vi "Load Configuration.vi"(8 "error in":errorcluster) -> (0 "error out":errorcluster, 3 "Theme Config out":refnum<class "Theme Config.lvclass">)   [LabVIEW 2021, in "Theme Config.lvclass"]
doc: "Load the configuration from file; if it doesn't exist, go ahead and create it so it can be referenced in the future.\n\nThis will allow persistence of the Material File in the editor and the Last Theme Mod implemented.\n\n<b>Code Developed By:</b>\nDaniel Coons\nTechnology Service Corporation\nwww.tsc.com/atcs"
uses:
  Theme Config.lvclass
  C:/Program Files/National Instruments/LabVIEW 2026/vi.lib/JDP Science/JSONtext/Config Files/Config File.lvclass
  Theme Serializer/Theme Serializer.lvclass
  C:/Program Files/National Instruments/LabVIEW 2026/vi.lib/JDP Science/JSONtext/LVClass Serializer/JSONtext LVClass Serializer.lvclass
  Theme Config.lvclass/Theme Config.ctl
  <vilib>/JDP Science/JSONtext/Config Files/Config File.lvclass/Config File.ctl
  3b317bd2-2840-4331-bfb7-99d377f3c52f.vi
  <vilib>/JDP Science/JSONtext/JSON text to Variant.vi
  <vilib>/JDP Science/JSONtext/Config Files/Config File.lvclass
  <vilib>/JDP Science/JSONtext/JSONtext.lvlib
  Material SubVIs/Material SubVIs.lvlib
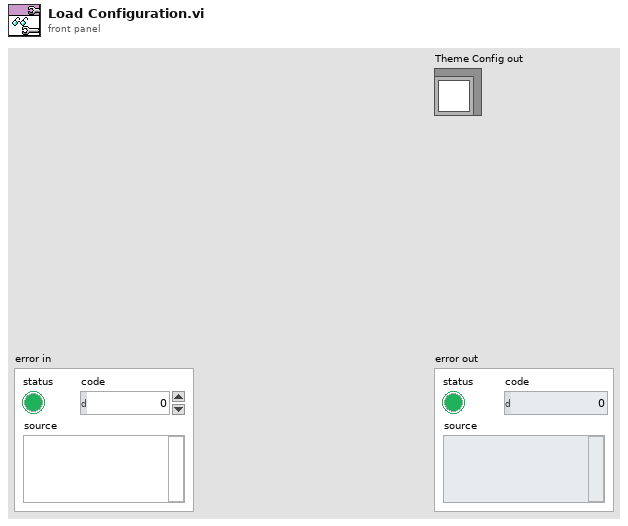
[diagram p1: front panel]
types:
  T1 = enum16{"open", "replace", "create", "open or create", "replace or create", "replace or create with confirmation"}
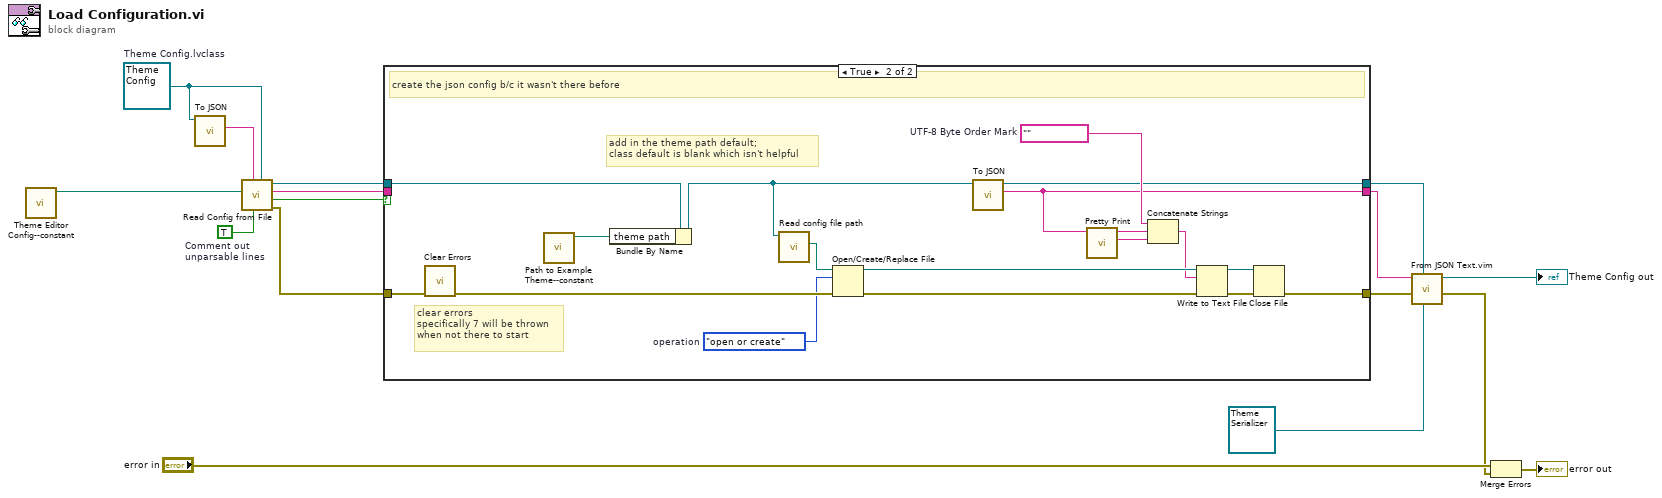
[diagram p0: block diagram]
diagram:
  w11 = TRUE  # Comment out unparsable lines
  w14 = refnum<class "Theme Config.lvclass"> refnum  # Theme Config.lvclass
  n1 = call "Theme Editor Config--constant.vi"() -> ("Button Editor Config"=w12:path)  [unwired: 11 in]
  n2 = call "To JSON.vi"("Theme Config in"=w14) -> ("JSON"=w13:string)  [unwired: 8 in, 2 out]
  n3 = call <vilib>:"Read Config from File.vi"("Config File (type)"=w14, "Comment out unparsable lines"=w11, "Template (JSON Object)"=w13, "config file path"=w12) -> ("error out"=w9:errorcluster, "Template Used (file missing or corrupted)"=w10:bool, "<JSON>Config"=w8:string, "Config File"=w7:refnum<class "Theme Config.lvclass">)  [unwired: 4 in]
  n4 = case shown="True" w10 {
    tunnel: w9 -> [w19 w37]
    tunnel: w8 -> [w18 _]
    tunnel: w7 -> [w17 w36]
    tunnel: [w17 w21] -> w4
    tunnel: [w18 w20] -> w5
    tunnel: [w19 w26] -> w6
    frame False {
    }
    frame True {
      w23 = T1."open or create"  # operation
      w30 = "﻿"  # UTF-8 Byte Order Mark
      # "add in the theme path default;\nclass default is blank which isn't helpful"
      # "clear errors\nspecifically 7 will be thrown\nwhen not there to start"
      # "create the json config b/c it wasn't there before"
      n5 = call <vilib>:"Clear Errors.vi"("error in (no error)"=w37) -> ("error out"=w24:errorcluster)  [unwired: 5 in, 1 out]
      n6 = call "Path to Example Theme--constant.vi"() -> ("Path to Example Theme"=w25:path)  [unwired: 11 in]
      n7 = Bundle By Name(cluster=w36, "theme path"=w25) -> (w22:refnum<class "Theme Config.lvclass">)
      n8 = call <vilib>:"Read config file path.vi"("Config File in"=w22) -> ("config file path"=w35:path)  [unwired: 10 in]
      n9 = Open/Create/Replace File(file path (use dialog)=w35, error in=w24, operation (0:open)=w23) -> (refnum out=w33:refnum<file>, error out=w34:errorcluster)  [unwired: 3 in, 1 out]
      n10 = call "To JSON.vi"("Theme Config in"=w22) -> ("JSON"=w20:string, "Theme Config out"=w21:refnum<class "Theme Config.lvclass">)  [unwired: 8 in, 1 out]
      n11 = call <vilib>:"Pretty Print.vi"("JSON"=w20) -> ("Rest of Input String"=w32:string, "<JSON>"=w31:string)  [unwired: 8 in, 1 out]
      n12 = Concatenate Strings(w30, w31, w32) -> (w29:string)
      n13 = Write to Text File(file (use dialog)=w33, text=w29, error in=w34) -> (refnum out=w27:refnum<file>, error out=w28:errorcluster)  [unwired: 1 in, 1 out]
      n14 = Close File(refnum=w27, error in=w28) -> (error out=w26:errorcluster)  [unwired: 1 out]
    }
  }
  n15 = call "From JSON Text.vim"("LVClass Serializer"=refnum<class "Theme Serializer.lvclass"> refnum ("Theme Serializer.lvclass"), "Data Type and Default Value"=w4, "error in (no error)"=w6, "JSON"=w5) -> ("error out"=w2:errorcluster, "Data out"=→"Theme Config out":refnum<class "Theme Config.lvclass">)  [unwired: 6 in]
  n16 = Merge Errors("error in", w2) -> (→"error out":errorcluster)
